vi "test_lugre_2.vi"() -> ()   [LabVIEW 2012]
uses:
  <vilib>/ptbypt/NI_PtbyPt.lvlib
panel:
  in  "stop":bool
  out "Waveform Chart":dbl(graph)
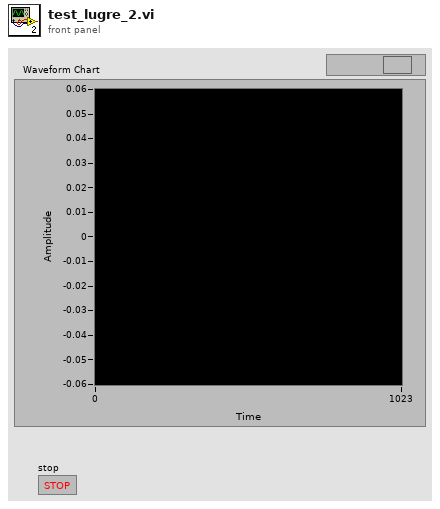
[diagram p1: front panel]
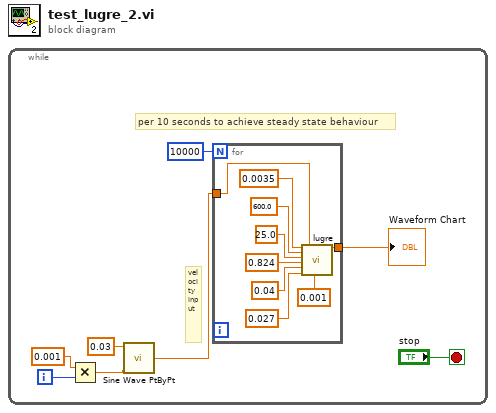
[diagram p0: block diagram]
diagram:
  n1 = while {
    i -> [w7]
    stop <- "stop" stop-if-true
    # "velocity input"
    # "per 10 seconds to achieve steady state behaviour"
    n2 = Multiply(x=0.001, y=w7) -> (x*y=w4:dbl)
    n3 = call <vilib>:"Sine Wave PtByPt.vi"("time"=w4, "amplitude"=0.03) -> ("sine wave"=w2:dbl)  [unwired: 2 in]
    n4 = for {
      N: 10000 -> [_]
      tunnel: w2 -> [w11]
      tunnel: [w10] -> w6
      n5 = call "lugre.vi"("stribeck velocity"=0.0035, "bristle stiffness"=600.0, "bristle damping"=25.0, "viscous friction"=0.824, "stiction friction"=0.04, "columb friction"=0.027, "velocity"=w11, "time sampling"=0.001) -> ("F"=w10:dbl)  [unwired: 10 in, 1 out]
    }
    "Waveform Chart" <- w6
  }
